vi "Building blocks.vi"() -> ()   [LabVIEW 2015]
uses:
  <vilib>/Analysis/Matrix/Datatypes/RealMatrix.ctl
  <vilib>/Platform/TimedLoop/XDataNode/timing_clust.ctl
  <vilib>/Platform/TimedLoop/XDataNode/nitl_modes.ctl
  <vilib>/Platform/TimedLoop/XDataNode/wakeup.ctl
  <vilib>/Analysis/2dsp.llb/Real FFT.vi
  <vilib>/imath/engines/lvmath2/RunTimeEngine/Managers/WorkSpace/UID Generator.vi
  <vilib>/Analysis/Matrix/Numeric/Conversions/Matrix To Array - RM.vi
  <vilib>/imath/engines/lvmath2/RunTimeEngine/IndexRead/NIMS M(S).vi
  <instcachedir>/0/NIMS M(S)_B826C018497E4940AE96BD27B540B6FB.lvgen/NIMS M(S)_B826C018497E4940AE96BD27B540B6FB_000.vi
  <vilib>/imathl/engines/lvmath/Functions/Error Handling/Create Error.vi
  <vilib>/imath/engines/lvmath2/RunTimeEngine/RunTimeType/NIMS_RunTimeType_From StrictType (excl LVString).vi
  <instcachedir>/0/NIMS_RunTimeType_From StrictType (excl LVString)_EB1C38A9BC5048DA9ABDA8F781E54D21.lvgen/NIMS_RunTimeType_From StrictType (excl LVString)_EB1C38A9BC5048DA9ABDA8F781E54D21_000.vi
  <vilib>/imath/engines/lvmath2/RunTimeEngine/LocalVariableDefStatement/MC_LocalVariableDefStatement_Display.vi
  <vilib>/imath/engines/lvmath2/RunTimeEngine/BuiltInFunctions/mod/NIMS_mod_no_size_check.vi
  <instcachedir>/0/NIMS_mod_no_size_check_5393E3382FD241D281EEB71DA286C65B.lvgen/NIMS_mod_no_size_check_5393E3382FD241D281EEB71DA286C65B_001.vi
  <vilib>/imath/engines/lvmath2/RunTimeSupport/NIMS_Complex To Real.vi
  <instcachedir>/0/NIMS_Complex To Real_01315F44AA8B4CE79FEF95AE999DC25E.lvgen/NIMS_Complex To Real_01315F44AA8B4CE79FEF95AE999DC25E_001.vi
  <vilib>/imath/engines/lvmath2/RunTimeEngine/BuiltInFunctions/atan/NIMS_atan(C).vi
  <instcachedir>/0/NIMS_atan(C)_2E5E67C8FA77440CAA2E5F1DC65089FF.lvgen/NIMS_atan(C)_2E5E67C8FA77440CAA2E5F1DC65089FF_001.vi
  <vilib>/imath/engines/lvmath2/RunTimeEngine/BuiltInFunctions/cos/NIMS_cos(C).vi
  <instcachedir>/0/NIMS_cos(C)_840A8FDA839D4E2AADB43697F53F61ED.lvgen/NIMS_cos(C)_840A8FDA839D4E2AADB43697F53F61ED_001.vi
  <vilib>/imath/engines/lvmath2/RunTimeEngine/Managers/SymbolTable/Clear UID.vi
  <vilib>/imath/engines/lvmath2/RunTimeEngine/NodeEndStatement/NIMS_NodeEndStatement_Output.vi
  <instcachedir>/0/NIMS_NodeEndStatement_Output_53EC0D466D134D7ABD903AC30B43404B.lvgen/NIMS_NodeEndStatement_Output_53EC0D466D134D7ABD903AC30B43404B_012.vi
  <instcachedir>/0/NIMS_NodeEndStatement_Output_53EC0D466D134D7ABD903AC30B43404B.lvgen/NIMS_NodeEndStatement_Output_53EC0D466D134D7ABD903AC30B43404B_009.vi
  <instcachedir>/0/NIMS_NodeEndStatement_Output_53EC0D466D134D7ABD903AC30B43404B.lvgen/NIMS_NodeEndStatement_Output_53EC0D466D134D7ABD903AC30B43404B_001.vi
  <vilib>/imath/engines/lvmath2/RunTimeEngine/ErrorHandling/NIMS_Finalize Error.vi
  <vilib>/Platform/TimedLoop/XDataNode/XDataNode.xnode
  <vilib>/Platform/TimedLoop/XDataNode/XDNodeRunTimeDep.lvlib
  <vilib>/Analysis/Matrix/NI_Matrix.lvlib
  <vilib>/imath/engines/lvmath2/RunTimeEngine/Managers/SymbolTable/NIMS_WorkSpace.lvlib
  <vilib>/Analysis/NI_AALPro.lvlib
panel:
  in  "?":enum32{"Monitoring", "Configuration"}(tab)
  in  "?":refnum<k7>(container)
  out "Azimuth (deg)":dbl format="%#_13g"
  out "Elevation (deg)":dbl format="%#_13g"
  out "Satellite's coordinates (ECI) (km)":T1
  out "Message":string
  out "Closed Link budget":bool
  out "Power Spectrum":cluster{"Elevation":sgl, dbl, dbl[]}(graph)
  in  "stop":bool
  in  "BW":i32
  in  "EIRPground (dBW)":dbl=2.0
  in  "Uplink frequency (MHz)":dbl=480.0 format="%#_13g"
  in  "Downlink frequency (MHz)":dbl=380.0 format="%#_13g"
  in  "G/Tsat (dBK-1)":dbl=10.0 format="%#_13g"
  in  "EIRPsat(dBW)":dbl=20.0 format="%#_13g"
  in  "G/T ground (dBK-1)":dbl=5.0 format="%#_13g"
  in  "Bandwidth (MHz)":dbl=36.0
  in  "Chosen Modulation":string(combo)
  in  "Bit rate (bits/s)":dbl=400000.0
  in  "Minimum margin (dB)":dbl=4.0 format="%#_13g"
  in  "TLE - Add the two last lines":string="1 33591U 09005A   15349.50189518  .00000223  00000-0  14631-3 0  9999\n2 33591  99.0150 300.0232 0014480  22.8695 337.3118 14.12015716353078"
  in  "Antenna latitude (°)":dbl
  in  "Antenna altitude (km)":dbl
  in  "Antenna east longitude (°)":dbl
  in  "Current UTC hour of the computer":dbl
  out "C/N0 (dBHz) required":dbl
  out "C/N (dBHz) required":dbl
  out "C/N0 uplink (dBHz)":dbl format="%#_13g"
  out "C/N0 downlink (dBHz)":dbl format="%#_13g"
  out "Margin (dB)":dbl
  out "C/N (dB)":dbl
  out "C/N0 tot (dBHz)":dbl format="%#_13g"
  in  "device name":refnum<k15>="192.168.10.2"
  in  "IQ Sampling\nRate [S/sec]":dbl=200000.0 format="%#.6p"
  in  "Carrier\nFrequency [Hz]":dbl=90500000.0 format="%#.6p"
  in  "Gain [dB]":dbl=20.0 format="%#.6p"
  in  "Active Antenna":string(combo)="RX1"
  # "SATELLITE INFORMATION"
  # "LINK BUDGET"
  # "SATELLITE CONFIGURATION"
  # "LINK CONFIGURATION"
  # "USRP CONFIGURATION"
  # "GROUND STATION CONFIGURATION"
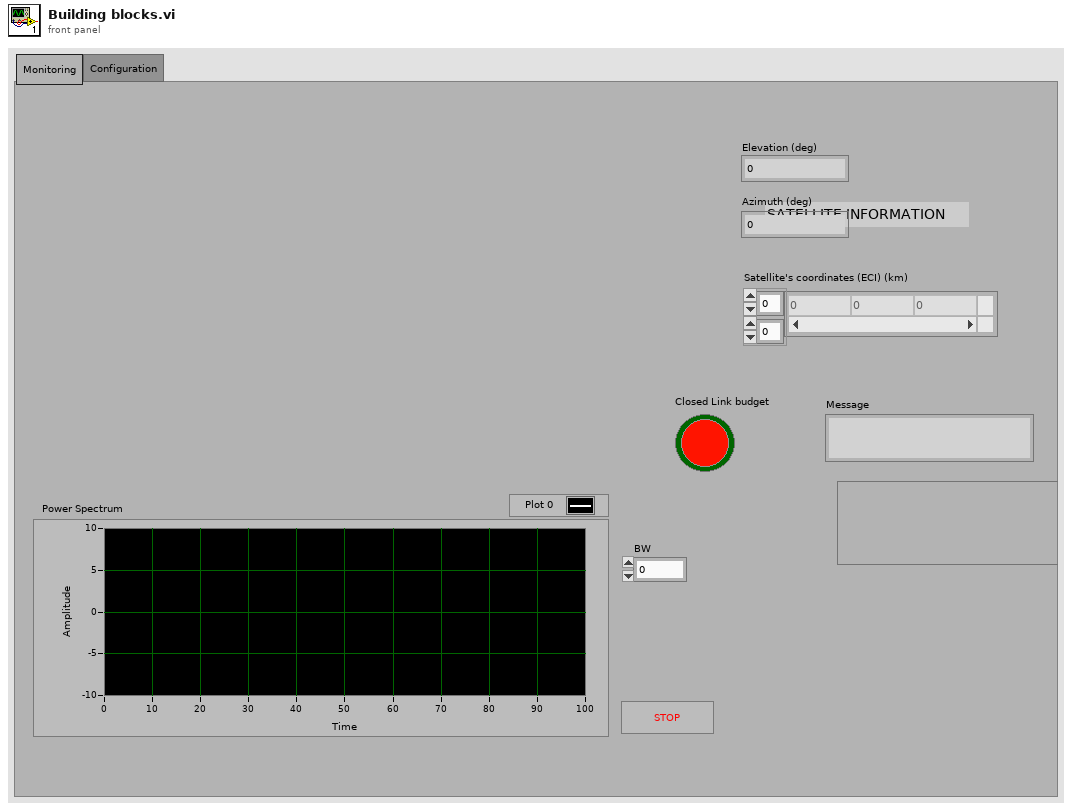
[diagram p1: front panel]
types:
  T1 = typedef "NI_Matrix.lvlib/RealMatrix.ctl" = dbl[][]
  T2 = typedef "XDNodeRunTimeDep.lvlib/timing_clust.ctl" = cluster{"Expected End [f-1]":u64, "Actual End [f-1]":u64, "Finished Late? [f-1]":bool, "Expected End [i-1]":u64, "Actual End [i-1]":u64, "Finished Late? [i-1]":bool, "Expected Start [i]":u64, "Actual Start [i]":u64, "Expected Start [f]":u64, "Actual Start [f]":u64, "Source Name":string, "Structure Name":string, "Period":i64, "Deadline":i64, "Offset":i64, "Start":i64, "Priority":i32, "Timeout":i32, "Mode":T3, "Wakeup Reason":T4, "Error":errorcluster, "Source Type":string, "Secondary Source Type":string, "Global End Time":u64, "Global Start Time":u64, "Frame Duration":u64, "Iteration Duration":u64, "Assigned CPU":i32, "I/O Scan Engine Mode":u32}
  T3 = typedef "XDNodeRunTimeDep.lvlib/nitl_modes.ctl" = enum32{"No Change", "Process missed periods, maintain original phase", "Discard missed periods, maintain original phase", "Process missed periods, ignore original phase", "Discard missed periods, ignore original phase"}
  T4 = typedef "XDNodeRunTimeDep.lvlib/wakeup.ctl" = enum32{"Normal", "Aborted", "Asynchronous wakeup", "Timing source error", "Timed loop error", "Timeout"}
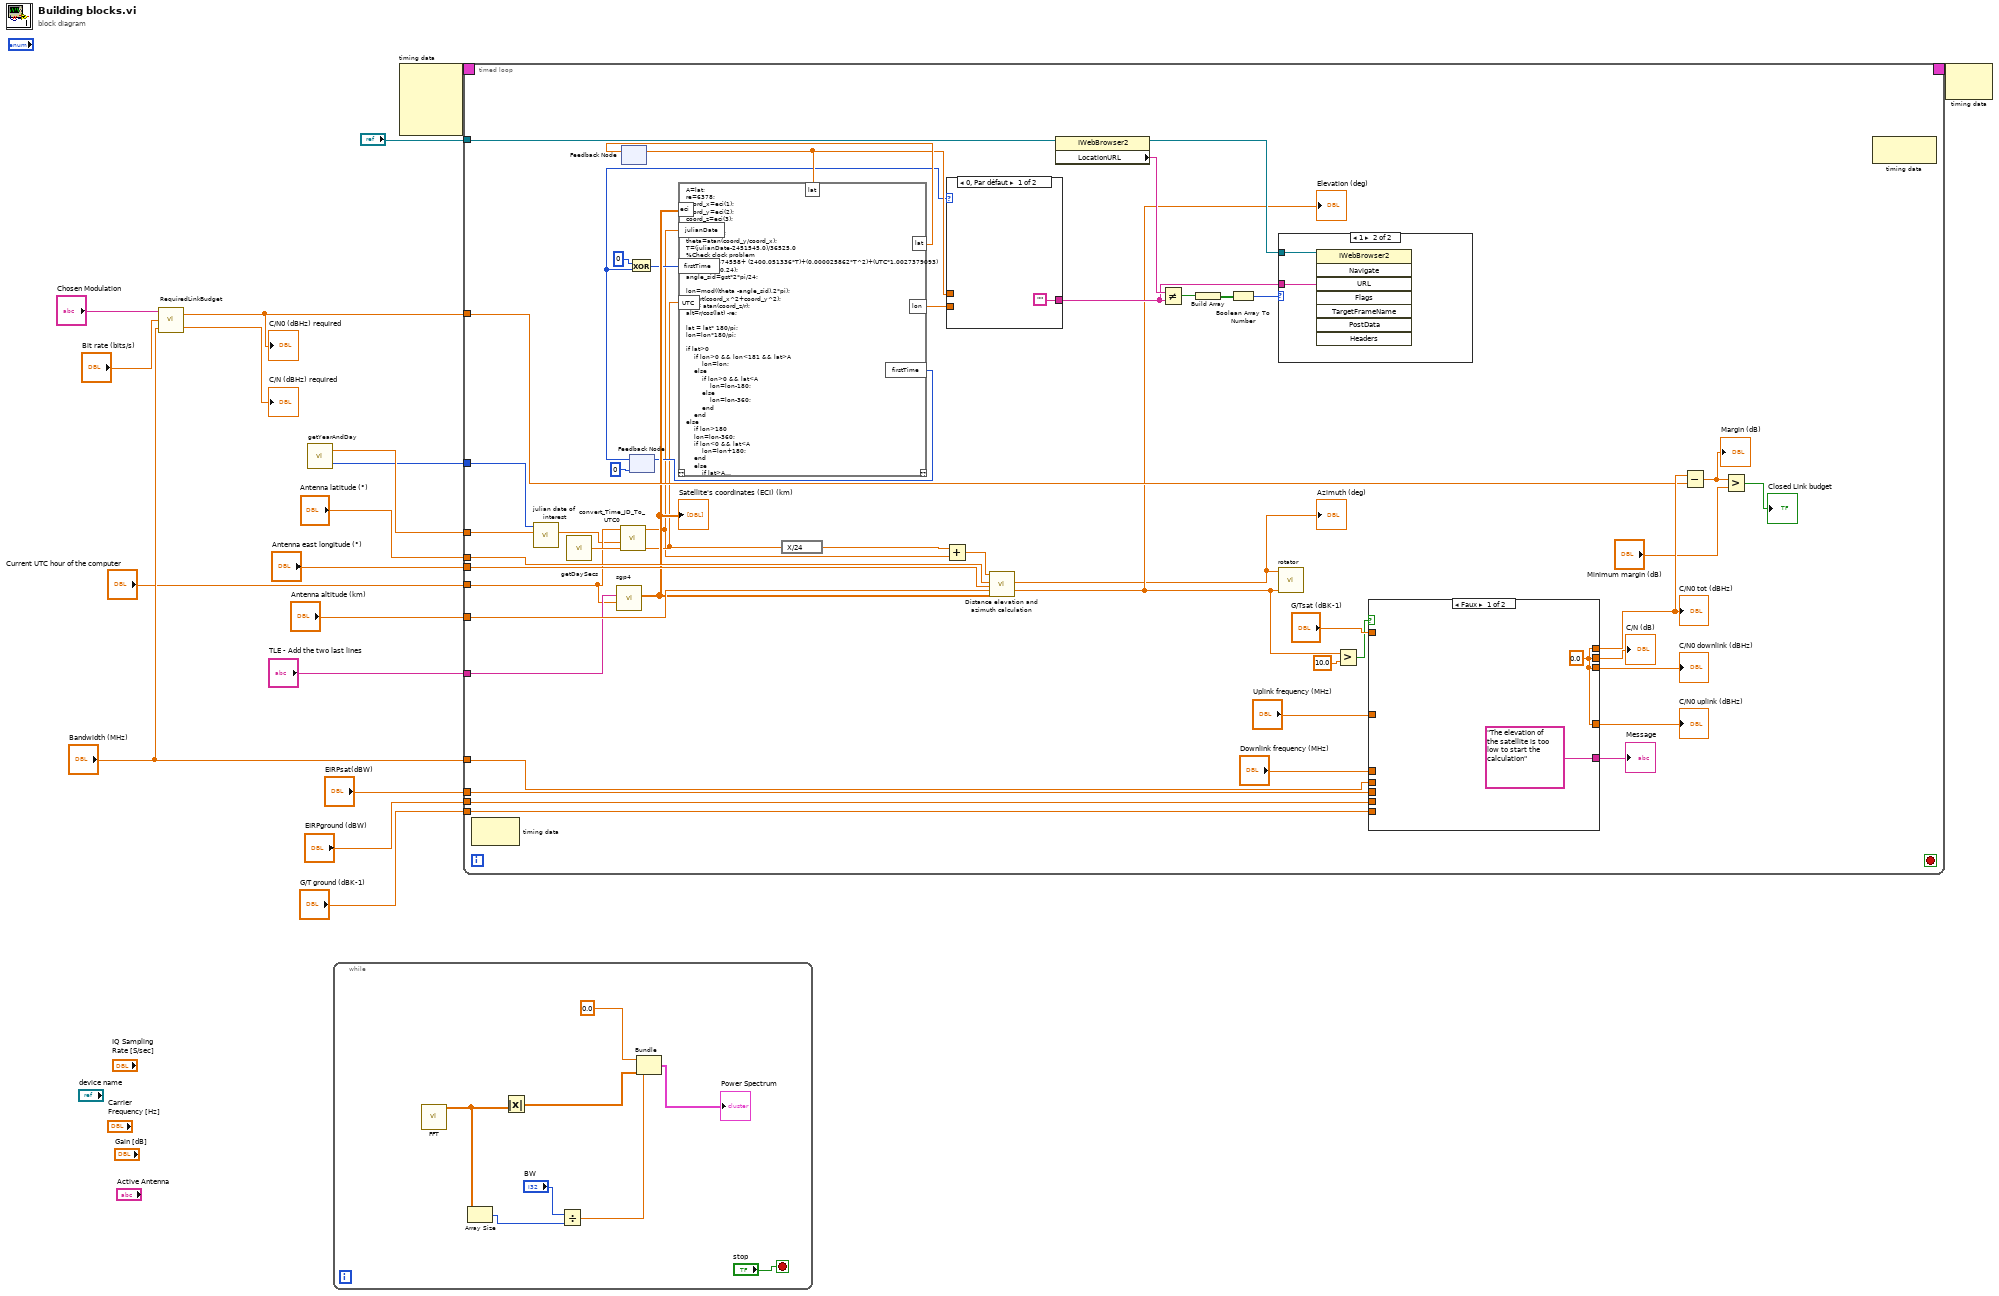
[diagram p0: block diagram]
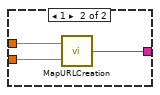
[diagram p2: hidden frame]
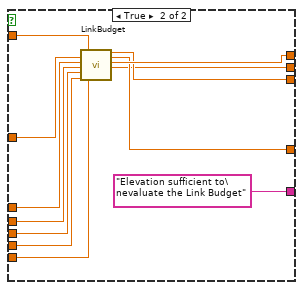
[diagram p4: hidden frame]
diagram:
  n1 = call "RequiredLinkBudget.vi"("Bandwith (MHz)"="Bandwidth (MHz)", "Bit rate (bits/s)"="Bit rate (bits/s)", "Chosen Modulation"="Chosen Modulation") -> ("C/N (dB) required"=→"C/N (dBHz) required":dbl, "C/N0 (dB) required"=w10:dbl)
  "C/N0 (dBHz) required" <- w10
  n2 = call "getYearAndDay.vi"() -> ("year"=w7:i32, "Day of the year"=w8:dbl)  [unwired: 2 in]
  n3 = while {
    stop <- "stop" stop-if-true
    n4 = call-poly <vilib>:"FFT.vi"() -> ("FFT {X}"=w20:cdb[])  [unwired: 10 in, 1 out]
    n5 = Array Size(array=w20) -> (size(s)=w21:i32)
    n6 = Absolute Value(x=w20) -> (abs(x)=w23:dbl[])
    n7 = Divide(x="BW", y=w21) -> (x/y=w24:dbl)
    n8 = Bundle("Elevation"=sgl 0.0, w24, w23) -> (→"Power Spectrum":cluster{"Elevation":sgl, dbl, dbl[]})  [unwired: 1 in]
  }
  n9 = node-c288() -> (w4:T2)  [unwired: 4 in]
  n10 = timed-loop {
    timing: w4 -> [_]
    timing-out: [_] -> w3
    tunnel: "EIRPsat(dBW)" -> [w75]
    tunnel: "G/T ground (dBK-1)" -> [w74]
    tunnel: "Antenna latitude (°)" -> [w73]
    tunnel: "Antenna east longitude (°)" -> [w72]
    tunnel: "Antenna altitude (km)" -> [w71]
    tunnel: w10 -> [w69]
    tunnel: "TLE - Add the two last lines" -> [w54]
    tunnel: w8 -> [w46]
    tunnel: w7 -> [w34]
    tunnel: "Bandwidth (MHz)" -> [w58]
    tunnel: "EIRPground (dBW)" -> [w57]
    tunnel: "?" -> [w48]
    tunnel: "Current UTC hour of the computer" -> [w40]
    stop <- _ stop-if-true
    n11 = node-c288() -> ()  [unwired: 1 in, 1 out]
    n12 = call "julian date of interest.vi"("Day of the year"=w46, "Year"=w34) -> ("Julian date of the day"=w33:dbl)  [unwired: 8 in, 1 out]
    n13 = call "getDaySecs.vi"() -> ("x+y"=w41:dbl)
    n14 = call "sgp4.vi"("UTC"=w40, "TLE"=w54) -> ("r"=w47:T1)  [unwired: 5 in]
    "Satellite's coordinates (ECI) (km)" <- w47
    n15 = call "convert_Time_JD_To_UTC0.vi"("ut_Sec"=w41, "Julian Date"=w33, "UTC"=w40) -> ("UTC+0"=w31:dbl, "Julian Date"=w30:dbl)  [unwired: 7 in]
    n16 = feedback #1() -> (w42:cdb)  [unwired: 1 in]
    n17 = feedback #2(0) -> (w37:i32)
    n18 = Exclusive Or(1:w37, 2:0) -> (0:w38:i32)
    n19 = mathscript code="A=lat; \nre=6378;\ncoord_x=eci(1);\ncoord_y=eci(2);\ncoord_z=eci(3);\n\n firstTime=1;\ntheta=atan(coord_y/coord_x);\nT=(julianDate-2451545.0)/36525.0\n%Check clock problem\nT0=6.697374558+ (2400.051336*T)+(0.000025862*T^2)+(UTC*1.0027379093)\ngst=mod(T0,24);\nangle_sid=gst*2*pi/24;\n\nlon=mod((theta -angle_sid),2*pi);\nr=sqrt(coord_x^2+coord_y^2);\nlat = atan(coord_z/r);\nalt=r/cos(lat) -re;\n \nlat = lat* 180/pi;\nlon=lon*180/pi;\n\nif lat>0\n    if lon>0 && lon<181 && lat>A\n        lon=lon;\n    else\n        if lon>0 && lat<A\n            lon=lon-180;\n        else\n            lon=lon-360;\n        end\n    end\nelse\n    if lon>180\n    lon=lon-360;\n    if lon<0 && lat<A\n        lon=lon+180;\n    end\n    else\n        if lat>A\n         lon=lon;\n        elseif lat<A\n            lon=lon-180;\n        end\n    end\nend" ("Nœud MathScript")("eci"=w47, "julianDate"=w30, "UTC"=w31, "lat"=w42, "firstTime"=w38) -> ("lat"=w43:cdb, "lon"=w45:dbl, "firstTime"=w36:i32)  [unwired: 1 in, 1 out]
    n20 = feedback-in #1(w43) -> ()
    n21 = feedback-in #2(w36) -> ()
    n22 = expression code="X/24"(w31) -> (w32:dbl)
    n23 = Add(x=w32, y=w30) -> (x+y=w29:dbl)
    n24 = case shown="0, Par défaut" w37 {
      tunnel: w45 -> [_ w79]
      tunnel: ["" w78] -> w44
      tunnel: w42 -> [_ w77]
      frame 0, Default {
      }
      frame 1 {
        n25 = call "MapURLCreation.vi"("Longitude"=w79, "Latitude"=w77) -> ("URL"=w78:string)
      }
    }
    n26 = call "Distance elevation and azimuth calculation.vi"("Julian Date"=w29, "Antenna latitude (°)"=w73, "Antenna east longitude (°)"=w72, "Antenna altitude (km)"=w71, "Position Satellite coordinate (ECI)"=w47) -> ("Azimuth (deg)"=w27:dbl, "Elevation (deg)"=w28:dbl)  [unwired: 13 in]
    "Azimuth (deg)" <- w27
    "Elevation (deg)" <- w28
    n27 = property class="IWebBrowser2"(reference=w48) -> (reference out=w53:refnum<k7>, "LocationURL"=w51:string)  [unwired: 1 in, 1 out]
    n28 = Not Equal?(x=w51, y=w44) -> (x != y?=w52:bool)
    n29 = Build Array(w52) -> (w50:bool[])
    n30 = Boolean Array To Number(Boolean array=w50) -> (number=w49:u32)
    n31 = case shown="1" w49 {
      tunnel: w44 -> [_ w530]
      tunnel: w53 -> [_ w529]
      frame 0, Default {
      }
      frame 1 {
        n32 = invoke class="IWebBrowser2" method="Navigate"(reference=w529, "URL"=w530) -> ()  [unwired: 6 in, 8 out]
      }
    }
    n33 = call "rotator.vi"("Elevation"=w28, "Azimuth"=w27) -> ()  [unwired: 10 in]
    n34 = Greater?(x=w28, y=10.0) -> (0:w59:bool)
    n35 = case shown="Faux" w59 {
      tunnel: w75 -> [_ w544]
      tunnel: w74 -> [_ w543]
      tunnel: w58 -> [_ w542]
      tunnel: [w532 w541] -> w70
      tunnel: "G/Tsat (dBK-1)" -> [_ w540]
      tunnel: "Uplink frequency (MHz)" -> [_ w539]
      tunnel: "Downlink frequency (MHz)" -> [_ w538]
      tunnel: [w532 w537] -> w63
      tunnel: [w532 w536] -> w62
      tunnel: [w532 w535] -> w61
      tunnel: w57 -> [_ w534]
      tunnel: ["The elevation of the satellite is too low to start the calculation" "Elevation sufficient to\nevaluate the Link Budget"] -> w56
      frame False {
        w532 = 0.0
      }
      frame True {
        n36 = call "LinkBudget.vi"("Uplink frequency (GHz)"=w539, "Downlink frequency (GHz)"=w538, "Bandwith (MHz)"=w542, "EIRPsat(dBW)"=w544, "EIRPground (dBW)"=w534, "G/Tsat (dB)"=w540, "G/T ground (dBK-1)"=w543) -> ("C/N0 downlink (dBHz)"=w537:dbl, "C/N0 uplink (dBHz)"=w536:dbl, "C/N0 tot (dB)"=w541:dbl, "C/N (dB)"=w535:dbl)  [unwired: 9 in]
      }
    }
    "C/N0 uplink (dBHz)" <- w62
    "C/N0 downlink (dBHz)" <- w63
    "C/N (dB)" <- w61
    "C/N0 tot (dBHz)" <- w70
    "Message" <- w56
    n37 = Subtract(x=w70, y=w69) -> (x-y=w68:dbl)
    "Margin (dB)" <- w68
    n38 = Greater?(x=w68, y="Minimum margin (dB)") -> (0:→"Closed Link budget":bool)
    n39 = node-c288() -> ()  [unwired: 1 in, 1 out]
  }
  n40 = node-c288(w3) -> ()  [unwired: 1 out]
